vi "Tracking Initialization.vi"(4 "Eye Model Cluster":T2={"X Grid"=[], "Y Grid"=[], "Za_true Surf"=[], "Iris Center"=[], "Zp_true Surf"=[], "Pinv"=[[1.0, 0.0], [0.0, 1.0]], "za_true"=5.0, "za_work"=1.0, "zp_work"=-1.0, "zp_true"=-5.0}, 5 "Trajectory Cluster":T3, 6 "PID Cluster":T5={"L1 to L4 PID Cluster"={"L1 PID Gains"={"Kp"=0.005, "Kd"=0.5, "Ki"=0.0005}, "L2 PID Gains"={"Kp"=0.01, "Kd"=1.0, "Ki"=0.005}, "L3 PID Gains"={"Kp"=0.05, "Kd"=1.0, "Ki"=0.0005}, "L4 PID Gains"={"Kp"=0.1, "Kd"=0.1, "Ki"=0.0005}}, "Stage PID Cluster"={"Stage Z PID"={"Kp"=0.0005, "Kd"=0.001, "Ki"=0.0}, "Stage Y PID"={"Kp"=0.0003, "Kd"=0.01, "Ki"=0.0}, "Stage X PID"={"Kp"=0.0003, "Kd"=0.01, "Ki"=0.0}}, "OCT Z PID Gains"={"Kp"=0.0003, "Kd"=0.0001, "Ki"=0.01}}, 7 "Offset Home 2 RCM":dbl[](array[numeric])=[0.0, 0.0, 0.0, 0.0], 8 "error in":errorcluster, 9 "Prev Index":i32, 10 "Prev Posit Cluster":T6={"Prev L1 to L4 Posit"=[0.0, 0.0, 0.0, 0.0], "Prev Stage Posit"=[6.0, 6.0, 6.0], "Prev OCT Z Posit"=0.0}, 11 "FPGA VI Reference In":refnum<k20>) -> (0 "error out":errorcluster, 1 "Last Index":i32, 2 "Last Posit Cluster":T4={"Last L1 to L4 Posit"=[0.0, 0.0, 0.0, 0.0], "Last Stage Posit"=[6.0, 6.0, 6.0], "Last OCT Z Posit"=0.0}, 3 "FPGA VI Reference Out":refnum<k20>)   [LabVIEW 2016]
uses:
  <vilib>/Analysis/Matrix/Datatypes/RealMatrix.ctl
  <vilib>/Platform/TimedLoop/XDataNode/timing_clust.ctl
  <vilib>/Platform/TimedLoop/XDataNode/nitl_modes.ctl
  <vilib>/Platform/TimedLoop/XDataNode/wakeup.ctl
  Global Variables.vi
  <vilib>/platform/TimedLoop/XDataNode/XDataNode.xnode
  <vilib>/Platform/TimedLoop/XDataNode/XDNodeRunTimeDep.lvlib
  <vilib>/Analysis/Matrix/NI_Matrix.lvlib
panel:
  out "In Servo Loop":bool
  out "Indexing Finished?":bool
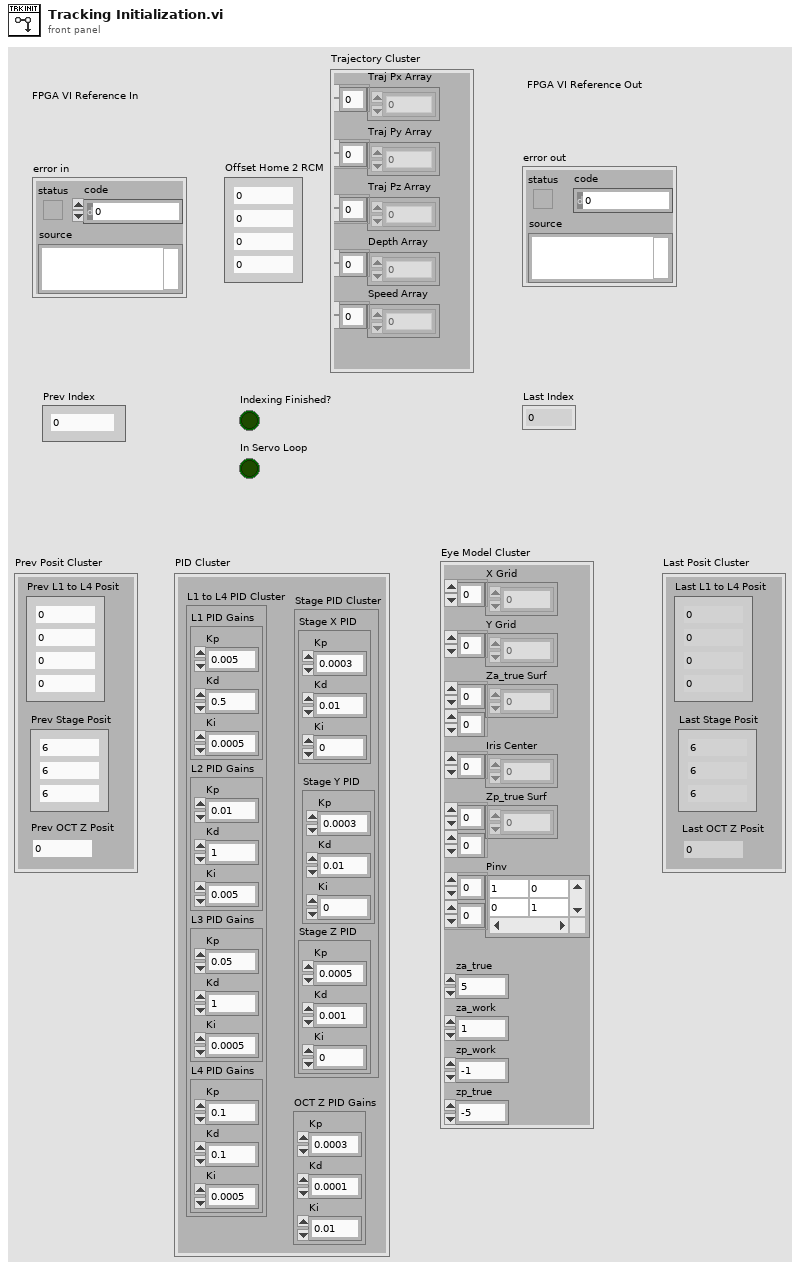
[diagram p1: front panel]
types:
  T1 = typedef "NI_Matrix.lvlib/RealMatrix.ctl" = dbl[][]
  T2 = cluster{"X Grid":dbl[], "Y Grid":dbl[], "Za_true Surf":dbl[][], "Iris Center":dbl[], "Zp_true Surf":dbl[][], "Pinv":T1, "za_true":dbl, "za_work":dbl, "zp_work":dbl, "zp_true":dbl}
  T3 = cluster{"Traj Px Array":dbl[], "Traj Py Array":dbl[], "Traj Pz Array":dbl[], "Speed Array":dbl[], "Depth Array":dbl[]}
  T4 = cluster{"Last L1 to L4 Posit":dbl[], "Last Stage Posit":dbl[], "Last OCT Z Posit":dbl}
  T5 = cluster{"L1 to L4 PID Cluster":cluster{"L1 PID Gains":cluster{"Kp":dbl, "Kd":dbl, "Ki":dbl}, "L2 PID Gains":cluster{"Kp":dbl, "Kd":dbl, "Ki":dbl}, "L3 PID Gains":cluster{"Kp":dbl, "Kd":dbl, "Ki":dbl}, "L4 PID Gains":cluster{"Kp":dbl, "Kd":dbl, "Ki":dbl}}, "Stage PID Cluster":cluster{"Stage Z PID":cluster{"Kp":dbl, "Kd":dbl, "Ki":dbl}, "Stage Y PID":cluster{"Kp":dbl, "Kd":dbl, "Ki":dbl}, "Stage X PID":cluster{"Kp":dbl, "Kd":dbl, "Ki":dbl}}, "OCT Z PID Gains":cluster{"Kp":dbl, "Kd":dbl, "Ki":dbl}}
  T6 = cluster{"Prev L1 to L4 Posit":dbl[], "Prev Stage Posit":dbl[], "Prev OCT Z Posit":dbl}
  T7 = typedef "XDNodeRunTimeDep.lvlib/timing_clust.ctl" = cluster{"Expected End [f-1]":u64, "Actual End [f-1]":u64, "Finished Late? [f-1]":bool, "Expected End [i-1]":u64, "Actual End [i-1]":u64, "Finished Late? [i-1]":bool, "Expected Start [i]":u64, "Actual Start [i]":u64, "Expected Start [f]":u64, "Actual Start [f]":u64, "Source Name":string, "Structure Name":string, "Period":i64, "Deadline":i64, "Offset":i64, "Start":i64, "Priority":i32, "Timeout":i32, "Mode":T8, "Wakeup Reason":T9, "Error":errorcluster, "Source Type":string, "Secondary Source Type":string, "Global End Time":u64, "Global Start Time":u64, "Frame Duration":u64, "Iteration Duration":u64, "Assigned CPU":i32, "I/O Scan Engine Mode":u32}
  T8 = typedef "XDNodeRunTimeDep.lvlib/nitl_modes.ctl" = enum32{"No Change", "Process missed periods, maintain original phase", "Discard missed periods, maintain original phase", "Process missed periods, ignore original phase", "Discard missed periods, ignore original phase"}
  T9 = typedef "XDNodeRunTimeDep.lvlib/wakeup.ctl" = enum32{"Normal", "Aborted", "Asynchronous wakeup", "Timing source error", "Timed loop error", "Timeout"}
  T10 = cluster{"Stop Vacuum":bool, "Vacuum Force":i8, "Max Limit [mmHg]":dbl, "Slide in":i8, "Irrigation?":bool}
  T11 = cluster{"L1 PID Gains":cluster{"Kp":dbl, "Kd":dbl, "Ki":dbl}, "L2 PID Gains":cluster{"Kp":dbl, "Kd":dbl, "Ki":dbl}, "L3 PID Gains":cluster{"Kp":dbl, "Kd":dbl, "Ki":dbl}, "L4 PID Gains":cluster{"Kp":dbl, "Kd":dbl, "Ki":dbl}}
  T12 = cluster{"Stage Z PID":cluster{"Kp":dbl, "Kd":dbl, "Ki":dbl}, "Stage Y PID":cluster{"Kp":dbl, "Kd":dbl, "Ki":dbl}, "Stage X PID":cluster{"Kp":dbl, "Kd":dbl, "Ki":dbl}}
  T13 = cluster{"Accurus button":bool[], "Accurus engaged?":bool, "Vacuum Force":i32, "Accurus Ch. A Vout":dbl, "Accurus Ch. B Vout":dbl, "Irrigation engaged?":bool}
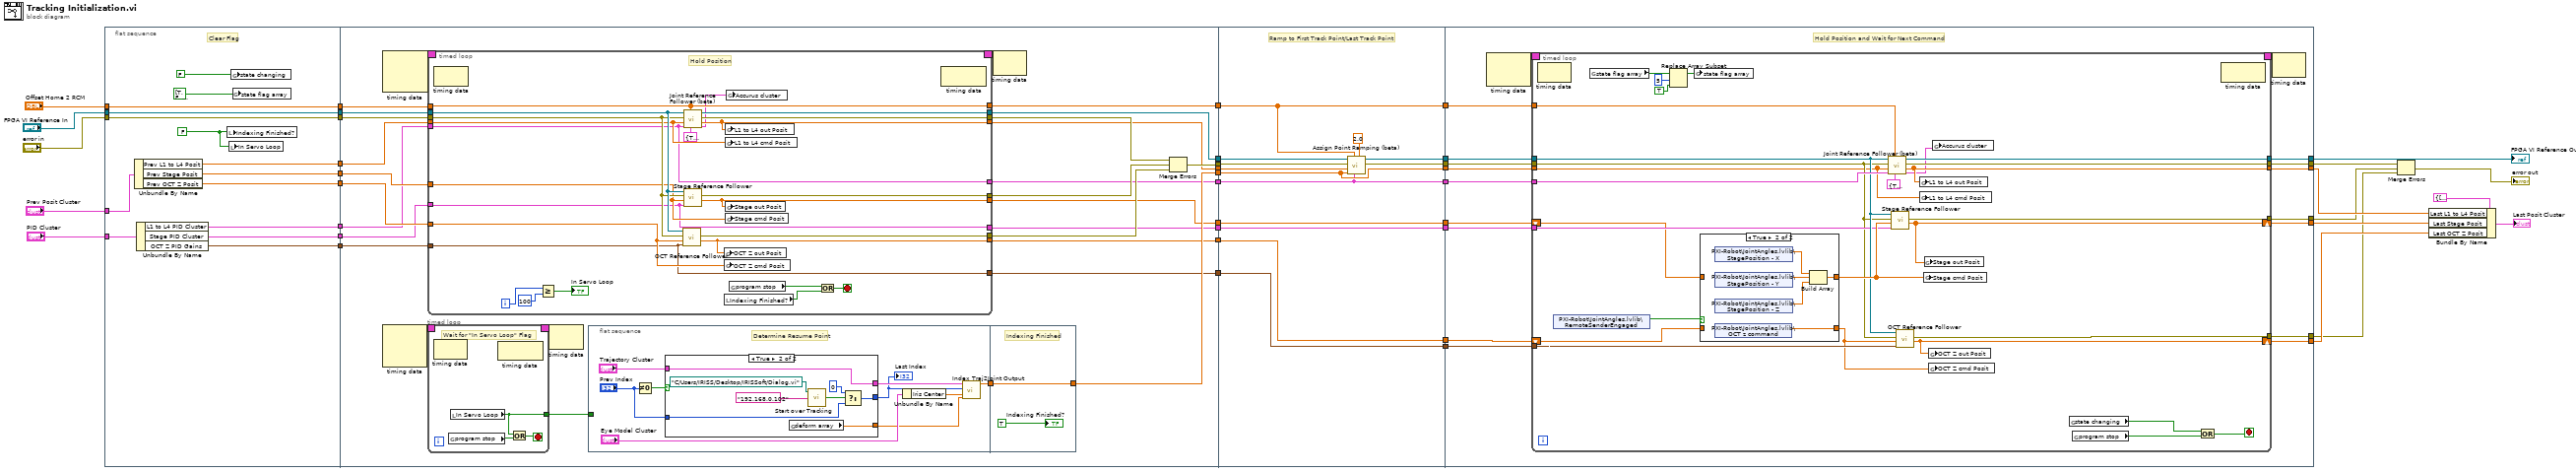
[diagram p0: block diagram]
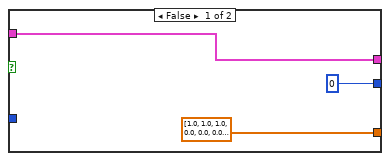
[diagram p2: hidden frame]
diagram:
  n1 = flat-sequence {
    tunnel: [w55] -> w21
    tunnel: "FPGA VI Reference In" -> [w55]
    tunnel: "error in" -> [w54]
    tunnel: [w54] -> w19
    tunnel: [w49] -> w17
    tunnel: "PID Cluster" -> [w48]
    tunnel: "Offset Home 2 RCM" -> [w53]
    tunnel: [w53] -> w15
    tunnel: "Prev Posit Cluster" -> [w52]
    tunnel: [w51] -> w12
    tunnel: [w50] -> w10
    tunnel: [w47] -> w8
    tunnel: [w46] -> w7
    tunnel: [w45] -> w6
    tunnel: w21 -> [w82]
    tunnel: [w76] -> w20
    tunnel: w19 -> [w81]
    tunnel: [w72] -> w18
    tunnel: w17 -> [w80]
    tunnel: [w71] -> w16
    tunnel: w15 -> [w83]
    tunnel: [w77] -> w14
    tunnel: [w70] -> w13
    tunnel: w12 -> [w79]
    tunnel: [w68] -> w11
    tunnel: w10 -> [w78]
    tunnel: [w69] -> w9
    tunnel: w8 -> [w67]
    tunnel: w7 -> [w66]
    tunnel: w6 -> [w65]
    tunnel: [w64] -> w5
    tunnel: [w63] -> w3
    tunnel: [w62] -> w1
    tunnel: w20 -> [w155]
    tunnel: w18 -> [w154]
    tunnel: w16 -> [w152]
    tunnel: w14 -> [w149]
    tunnel: w13 -> [w148]
    tunnel: [w151] -> w41
    tunnel: [w148] -> w40
    tunnel: [w150] -> w39
    tunnel: [w149] -> w38
    tunnel: [w145] -> w35
    tunnel: [w143] -> w34
    tunnel: w11 -> [w147]
    tunnel: [w147] -> w22
    tunnel: w9 -> [w144]
    tunnel: w5 -> [w146]
    tunnel: [w146] -> w4
    tunnel: w3 -> [w145]
    tunnel: [w144] -> w2
    tunnel: w1 -> [w143]
    tunnel: [w168] -> w30
    tunnel: [w167] -> w25
    tunnel: w41 -> [w170]
    tunnel: w40 -> [w157]
    tunnel: w39 -> [w171]
    tunnel: w38 -> [w158]
    tunnel: [w166] -> w36
    tunnel: [w165] -> w37
    tunnel: w35 -> [w164]
    tunnel: w34 -> [w163]
    tunnel: [w162] -> w31
    tunnel: [w161] -> w24
    tunnel: [w160] -> w23
    tunnel: w22 -> [w159]
    tunnel: w4 -> [w169]
    tunnel: w2 -> [w156]
    frame #0 {
      w44 = FALSE ("Indexing Finished?")
      # "Clear Flag"
      n2 = Unbundle By Name(w52) -> ("Prev L1 to L4 Posit"=w49:dbl[], "Prev Stage Posit"=w51:dbl[], "Prev OCT Z Posit"=w50:dbl)
      n3 = Unbundle By Name(w48) -> ("L1 to L4 PID Cluster"=w47:T11, "Stage PID Cluster"=w46:T12, "OCT Z PID Gains"=w45:cluster{"Kp":dbl, "Kd":dbl, "Ki":dbl})
      n4 = local write "Indexing Finished?"(w44) -> ()
      n5 = local write "In Servo Loop"(w44) -> ()
      n6 = global write "Global Variables.vi" "state changing"(FALSE ("state changing")) -> ()
      n7 = global write "Global Variables.vi" "state flag array"(bool[] [TRUE, FALSE, FALSE, FALSE, FALSE, FALSE, FALSE, FALSE, FALSE] ("state flag array")) -> ()
    }
    frame #1 {
      n8 = node-c288() -> (w61:T7)  [unwired: 3 in]
      n9 = node-c288() -> (w85:T7)  [unwired: 3 in]
      n10 = timed-loop {
        timing: w61 -> [_]
        timing-out: [_] -> w60
        tunnel: [w108] -> w59
        stop <- w110 stop-if-true
        # "Wait for \"In Servo Loop\" Flag"
        n11 = node-c288() -> ()  [unwired: 1 in, 1 out]
        n12 = global read "Global Variables.vi" "program stop"() -> (w109:bool)
        n13 = local read "In Servo Loop"() -> (w108:bool)
        n14 = node-c288() -> ()  [unwired: 1 in, 1 out]
        n15 = Or(x=w108, y=w109) -> (x .or. y?=w110:bool)
      }
      n16 = timed-loop {
        timing: w85 -> [_]
        timing-out: [_] -> w84
        tunnel: w83 -> [w133]
        tunnel: w82 -> [w138]
        tunnel: w81 -> [w137]
        tunnel: w80 -> [w136]
        tunnel: w79 -> [w135]
        tunnel: w78 -> [w134]
        tunnel: [w133] -> w77
        tunnel: [w132] -> w76
        tunnel: [w131] -> w75
        tunnel: [w130] -> w74
        tunnel: [w129] -> w73
        tunnel: [w128] -> w71
        tunnel: [w127] -> w68
        tunnel: [w126] -> w69
        tunnel: w67 -> [w122]
        tunnel: w66 -> [w121]
        tunnel: w65 -> [w120]
        tunnel: [w122] -> w64
        tunnel: [w121] -> w63
        tunnel: [w120] -> w62
        i -> [w119]
        stop <- w124 stop-if-true
        # "Hold Position"
        n17 = node-c288() -> ()  [unwired: 1 in, 1 out]
        n18 = Greater Or Equal?(x=w119, y=100) -> (x >= y?=→"In Servo Loop":bool)
        n19 = call "OCT Reference Follower.vi"("OCT Z PID Gains"=w120, "OCT  Z cmd Posit [mm]"=w134, "error in"=w137, "FPGA VI Reference In"=w138) -> ("OCT  Z out Posit [mm]"=w126:dbl, "error out"=w129:errorcluster)  [unwired: 5 in, 1 out]
        n20 = call "Joint Reference Follower (beta).vi"("Accurus Ctrl Cluster"=T10 {"Stop Vacuum"=TRUE, "Vacuum Force"=0, "Max Limit [mmHg]"=600.0, "Slide in"=0, "Irrigation?"=TRUE}, "Offset Home2RCM [deg/mm]"=w133, "PID Ctrl Cluster"=w122, "Ref Array [deg/mm]"=w136, "error in"=w137, "FPGA VI Reference In"=w138) -> ("Accurus Output Cluster"=w115:T13, "Output Posit Array [deg/mm]"=w128:dbl[], "error out"=w131:errorcluster, "FPGA VI Reference Out"=w132:refnum<k20>)  [unwired: 2 in]
        n21 = call "Stage Reference Follower.vi"("Stage PID Cluster"=w121, "Stage cmd Posit [mm]"=w135, "error in"=w137, "FPGA VI Reference In"=w138) -> ("Stage out Posit [mm]"=w127:dbl[], "error out"=w130:errorcluster)  [unwired: 5 in, 1 out]
        n22 = global write "Global Variables.vi" "OCT Z out Posit"(w126) -> ()
        n23 = global write "Global Variables.vi" "OCT Z cmd Posit"(w134) -> ()
        n24 = local read "Indexing Finished?"() -> (w123:bool)
        n25 = global write "Global Variables.vi" "L1 to L4 out Posit"(w128) -> ()
        n26 = global write "Global Variables.vi" "L1 to L4 cmd Posit"(w136) -> ()
        n27 = global write "Global Variables.vi" "Stage out Posit"(w127) -> ()
        n28 = global write "Global Variables.vi" "Stage cmd Posit"(w135) -> ()
        n29 = global write "Global Variables.vi" "Accurus cluster"(w115) -> ()
        n30 = global read "Global Variables.vi" "program stop"() -> (w125:bool)
        n31 = Or(x=w125, y=w123) -> (x .or. y?=w124:bool)
        n32 = node-c288() -> ()  [unwired: 1 in, 1 out]
      }
      n33 = node-c288(w60) -> ()  [unwired: 1 out]
      n34 = flat-sequence {
        tunnel: w59 -> [_]
        tunnel: [w87] -> w58
        tunnel: [w106] -> w70
        tunnel: w58 -> [w106]
        frame #0 {
          # "Determine Resume Point"
          n35 = Not Equal To 0?(x="Prev Index") -> (x != 0?=w94:bool)
          n36 = case shown="True" w94 {
            tunnel: [0 ("t") w104] -> w89
            tunnel: "Prev Index" -> [_ w103]
            tunnel: "Trajectory Cluster" -> [w96 w102]
            tunnel: [w96 w102] -> w91
            tunnel: [dbl[] [1.0, 1.0, 1.0, 0.0, 0.0, 0.0, 0.0, 0.0, 0.0] ("Deform Array") w98] -> w86
            frame False {
            }
            frame True {
              n37 = global read "Global Variables.vi" "deform array"() -> (w98:dbl[])
              n38 = call "Start over Tracking.vi"("Host System IP Address"="192.168.0.102", "VI Path on Host"=path "C:/Users/IRISS/Desktop/IRISSoft/Dialog.vi" ("vi path")) -> ("yes/no?"=w101:bool)  [unwired: 2 in, 1 out]
              n39 = Select(t=0, s=w101, f=w103) -> (s? t:f=w104:i32)
            }
          }
          "Last Index" <- w89
          n40 = Unbundle By Name("Eye Model Cluster") -> ("Iris Center"=w88:dbl[])
          n41 = call "Index Traj2Joint Output.vi"("Deform Array"=w86, "Pivot Pt"=w88, "Index"=w89, "Trajectory Cluster"=w91) -> ("Indexed Joit Posit"=w87:dbl[])  [unwired: 6 in, 1 out]
        }
        frame #1 {
          # "Indexing Finished"
          "Indexing Finished?" <- TRUE ("Indexing Finished?")
        }
      }
      n42 = node-c288(w84) -> ()  [unwired: 1 out]
      n43 = Merge Errors(w75, w74, w73) -> (w72:errorcluster)
    }
    frame #2 {
      # "Ramp to First Track Point/Last Track Point"
      n44 = call "Assign Point Ramping (beta).vi"("Ramp Time [sec]"=2.0, "L1 to L4 PID Cluster"=w146, "Offset Home2RCM"=w149, "Destination Posit Array [mm]"=w148, "Previous Posit Array"=w152, "error in"=w154, "FPGA VI Reference In"=w155) -> ("error out"=w151:errorcluster, "FPGA VI Reference Out"=w150:refnum<k20>)  [unwired: 2 in, 1 out]
    }
    frame #3 {
      # "Hold Position and Wait for Next Command"
      n45 = node-c288() -> (w173:T7)  [unwired: 2 in]
      n46 = timed-loop {
        timing: w173 -> [_]
        timing-out: [_] -> w172
        tunnel: w171 -> [w190]
        tunnel: w170 -> [w182]
        tunnel: w158 -> [w196]
        tunnel: w157 -> [w176]
        tunnel: w169 -> [w195]
        tunnel: [w194] -> w168
        tunnel: [w193] -> w167
        tunnel: [w188] -> w166
        tunnel: w164 -> [w187]
        tunnel: w163 -> [w186]
        tunnel: [w181] -> w161
        tunnel: [w180] -> w160
        shift-right: [w191] -> w165
        shift-left: w159 -> [w178]
        shift-right: [w185] -> w162
        shift-left: w156 -> [w177]
        stop <- w183 stop-if-true
        n47 = node-c288() -> ()  [unwired: 1 in, 1 out]
        n48 = shared-variable "PXI-Robot\\JointAngles.lvlib\\RemoteSenderEngaged"() -> (w179:bool)  [unwired: 1 in, 1 out]
        n49 = global read "Global Variables.vi" "state flag array"() -> (w200:bool[])
        n50 = Replace Array Subset(array=w200, new element=TRUE ("new element/subarray"), index=5) -> (w199:bool[])
        n51 = global write "Global Variables.vi" "state flag array"(w199) -> ()
        n52 = case shown="True" w179 {
          tunnel: [w203 w205] -> w192
          tunnel: [w202 w204] -> w184
          tunnel: w178 -> [w203 _]
          tunnel: w177 -> [w202 _]
          frame False {
            # "Hold Position if not Engaged"
          }
          frame True {
            n53 = shared-variable "PXI-Robot\\JointAngles.lvlib\\StagePosition - X"() -> (w208:dbl)  [unwired: 1 in, 1 out]
            n54 = shared-variable "PXI-Robot\\JointAngles.lvlib\\StagePosition - Y"() -> (w207:dbl)  [unwired: 1 in, 1 out]
            n55 = shared-variable "PXI-Robot\\JointAngles.lvlib\\StagePosition - Z"() -> (w206:dbl)  [unwired: 1 in, 1 out]
            n56 = shared-variable "PXI-Robot\\JointAngles.lvlib\\OCT z command"() -> (w204:dbl)  [unwired: 1 in, 1 out]
            n57 = Build Array(w208, w207, w206) -> (w205:dbl[])
          }
        }
        n58 = call "Joint Reference Follower (beta).vi"("Accurus Ctrl Cluster"=T10 {"Stop Vacuum"=TRUE, "Vacuum Force"=0, "Max Limit [mmHg]"=600.0, "Slide in"=0, "Irrigation?"=TRUE}, "Offset Home2RCM [deg/mm]"=w196, "PID Ctrl Cluster"=w195, "Ref Array [deg/mm]"=w176, "error in"=w182, "FPGA VI Reference In"=w190) -> ("Accurus Output Cluster"=w174:T13, "Output Posit Array [deg/mm]"=w188:dbl[], "error out"=w193:errorcluster, "FPGA VI Reference Out"=w194:refnum<k20>)  [unwired: 2 in]
        n59 = call "Stage Reference Follower.vi"("Stage PID Cluster"=w187, "Stage cmd Posit [mm]"=w192, "error in"=w182, "FPGA VI Reference In"=w190) -> ("Stage out Posit [mm]"=w191:dbl[], "error out"=w181:errorcluster)  [unwired: 5 in, 1 out]
        n60 = call "OCT Reference Follower.vi"("OCT Z PID Gains"=w186, "OCT  Z cmd Posit [mm]"=w184, "error in"=w182, "FPGA VI Reference In"=w190) -> ("OCT  Z out Posit [mm]"=w185:dbl, "error out"=w180:errorcluster)  [unwired: 5 in, 1 out]
        n61 = global write "Global Variables.vi" "L1 to L4 out Posit"(w188) -> ()
        n62 = global write "Global Variables.vi" "L1 to L4 cmd Posit"(w176) -> ()
        n63 = global write "Global Variables.vi" "Stage cmd Posit"(w192) -> ()
        n64 = global write "Global Variables.vi" "Stage out Posit"(w191) -> ()
        n65 = global write "Global Variables.vi" "OCT Z out Posit"(w185) -> ()
        n66 = global write "Global Variables.vi" "OCT Z cmd Posit"(w184) -> ()
        n67 = global write "Global Variables.vi" "Accurus cluster"(w174) -> ()
        n68 = global read "Global Variables.vi" "state changing"() -> (w201:bool)
        n69 = global read "Global Variables.vi" "program stop"() -> (w189:bool)
        n70 = Or(x=w201, y=w189) -> (x .or. y?=w183:bool)
        n71 = node-c288() -> ()  [unwired: 1 in, 1 out]
      }
      n72 = node-c288(w172) -> ()  [unwired: 1 out]
    }
  }
  n73 = Merge Errors(w25, w24, w23) -> (→"error out":errorcluster)
  n74 = Bundle By Name(cluster=T4 {"Last L1 to L4 Posit"=[0.0, 0.0, 0.0, 0.0], "Last Stage Posit"=[6.0, 6.0, 6.0], "Last OCT Z Posit"=0.0} ("Last Posit Cluster 2"), "Last L1 to L4 Posit"=w36, "Last Stage Posit"=w37, "Last OCT Z Posit"=w31) -> (→"Last Posit Cluster":T4)
  "FPGA VI Reference Out" <- w30
